vi "Triangle values.vi"(1 "Triangle Info":T1) -> (0 "Triangle Info Out":T1)   [LabVIEW 2012]
panel:
  # "Operator Info"
  # "R"
  # "L"
  # "Operator Info"
  # "R"
  # "L"
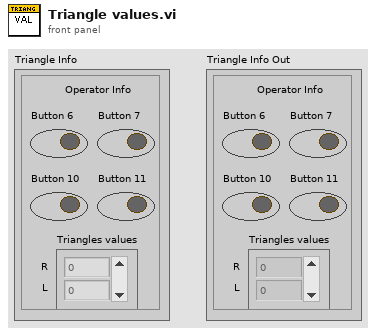
[diagram p1: front panel]
types:
  T1 = cluster{"Button 6":bool, "Button 7":bool, "Button 10":bool, "Button 11":bool, "Triangles values":dbl[]}
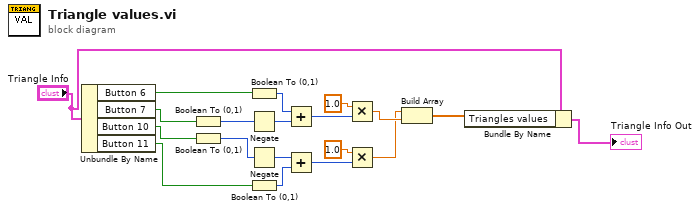
[diagram p0: block diagram]
diagram:
  n1 = Unbundle By Name("Triangle Info") -> ("Button 6"=w9:bool, "Button 7"=w8:bool, "Button 10"=w7:bool, "Button 11"=w6:bool)
  n2 = Boolean To (0,1)(Boolean=w8) -> (0, 1=w10:i16)
  n3 = Boolean To (0,1)(Boolean=w7) -> (0, 1=w19:i16)
  n4 = Boolean To (0,1)(Boolean=w9) -> (0, 1=w12:i16)
  n5 = Negate(x=w10) -> (-x=w11:i16)
  n6 = Negate(x=w19) -> (-x=w18:i16)
  n7 = Boolean To (0,1)(Boolean=w6) -> (0, 1=w17:i16)
  n8 = Add(x=w12, y=w11) -> (x+y=w13:i16)
  n9 = Add(x=w18, y=w17) -> (x+y=w16:i16)
  n10 = Multiply(x=1.0, y=w13) -> (x*y=w4:dbl)
  n11 = Multiply(x=1.0, y=w16) -> (x*y=w3:dbl)
  n12 = Build Array(w3, w4) -> (w2:dbl[])
  n13 = Bundle By Name(cluster="Triangle Info", "Triangles values"=w2) -> (→"Triangle Info Out":T1)
